vi "Get N Pin Objects.vi"(8 "error in":errorcluster, 10 "pin or relay names":string[](array[string]), 11 "session reservation in":refnum<class "Session Reservation.lvclass">) -> (0 "error out":errorcluster, 2 "instrument objects":refnum<class "DMM_Base.lvclass">[](array[class]), 3 "session reservation out":refnum<class "Session Reservation.lvclass">)   [LabVIEW 2021, in "DMM_Base.lvclass"]
doc: "Gets an array of pin_name and gives an array of LabVIEW object for given pins. The LabVIEW objects are then typecasted to the DMM_Base class objects and and each objects are updated with the session reservation, pin_name and the channel information."
uses:
  DMM_Base.lvclass
  <vilib>/Plug-In SDKs/Clients/Session Management V1/Session Reservation/Session Reservation.lvclass
  Reusables/Get Pin Information.lvlib
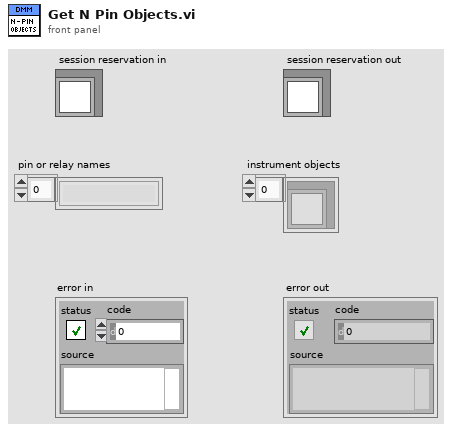
[diagram p1: front panel]
types:
  T1 = typedef "ni.measurementlink.sessionmanagement.v1.api.lvlib/ni_measurementlink_sessionmanagement_v1_ChannelMapping.ctl" = cluster{"pin_or_relay_name":string, "site":i32, "channel":string, "multiplexer_resource_name":string, "multiplexer_route":string}
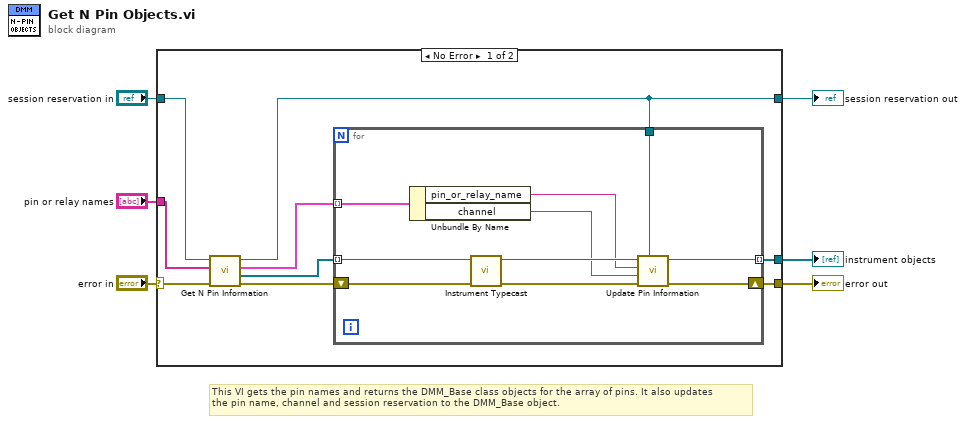
[diagram p0: block diagram]
diagram:
  # "This VI gets the pin names and returns the DMM_Base class objects for the array of pins. It also updates\nthe pin name, channel and session reservation to the DMM_Base object."
  n1 = case shown="No Error" "error in" {
    selector: "error in" -> [w13 w27]
    tunnel: "session reservation in" -> [w15 w26]
    tunnel: "pin or relay names" -> [w14 _]
    tunnel: [w9 _] -> w3
    tunnel: [w8 w27] -> w2
    tunnel: [w7 w26] -> w1
    frame No Error {
      n2 = call "Get N Pin Information.vi"("error in"=w13, "pin or relay names"=w14, "session reservation in"=w15) -> ("error out"=w10:errorcluster, "pin instruments"=w11:refnum<class>[], "channel_mappings"=w12:T1[], "session reservation out"=w7:refnum<class "Session Reservation.lvclass">)  [unwired: 5 in]
      n3 = for {
        tunnel: w12 -> [w25] mode=indexing
        tunnel: w11 -> [w16] mode=indexing
        shift-right: [w19] -> w8
        shift-left: w10 -> [w23]
        tunnel: [w18] -> w9 mode=indexing
        tunnel: w7 -> [w17]
        n4 = Unbundle By Name(w25) -> ("pin_or_relay_name"=w21:string, "channel"=w20:string)
        n5 = call "Instrument Typecast.vi"("error in (no error)"=w23, "pin instrument"=w16) -> ("error out"=w24:errorcluster, "instrument object"=w22:refnum<class "DMM_Base.lvclass">)  [unwired: 8 in]
        n6 = call "Update Pin Information.vi"("Session Reservation"=w17, "error in"=w24, "channel"=w20, "pin_name"=w21, "instrument object in"=w22) -> ("error out"=w19:errorcluster, "instrument object out"=w18:refnum<class "DMM_Base.lvclass">)  [unwired: 5 in]
      }
    }
    frame Error {
    }
  }
  "session reservation out" <- w1
  "instrument objects" <- w3
  "error out" <- w2
